vi "Get Result.vi"(8 "error in (no error)":errorcluster, 11 "Keithley Meter in":refnum<class "Keithley Meter.lvclass">) -> (0 "error out":errorcluster, 2 "Mag Lab Result.lvclass":refnum<class "Mag Lab Result.lvclass">, 3 "Keithley Meter out":refnum<class "Keithley Meter.lvclass">)   [LabVIEW 2015, in "Keithley Meter.lvclass"]
uses:
  Keithley Meter.lvclass
  Mag Lab Result/Mag Lab Result.lvclass
  Mag Lab Hardware.lvclass/Mag Lab Hardware.ctl
  Mag Lab Root/Mag Lab Root.lvclass/Mag Lab Root.ctl
  Keithley Meter.lvclass/Keithley Meter.ctl
  Instruments/Keithley/Meter/Keithley Meter Parameters.ctl
  Instruments/Keithley/Meter/KeithleyMeter Function.ctl
  Mag Lab Properties/Mag Lab Parameters.lvclass
  Mag Lab Hardware.lvclass
  Mag Lab Error Handler/Mag Lab Error Handler.lvclass
  Mag Lab Root/Mag Lab Root.lvclass
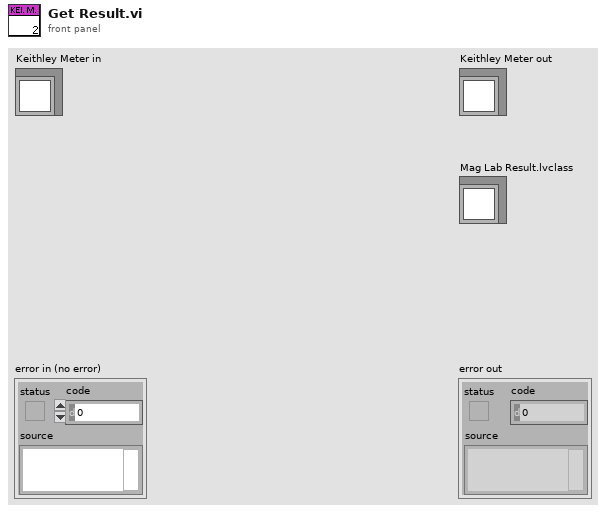
[diagram p1: front panel]
types:
  T1 = typedef "Keithley Meter Parameters.ctl" = cluster{"Range (-1: auto)":dbl, "Integration Time (NPLCs)":dbl, "Function":T2, "W Offset comp":bool, "4-wire W":bool, "Scale":dbl, "Offset":dbl}
  T2 = typedef "KeithleyMeter Function.ctl" = enum16{"VOLTAGE", "CURRENT", "RESISTANCE"}
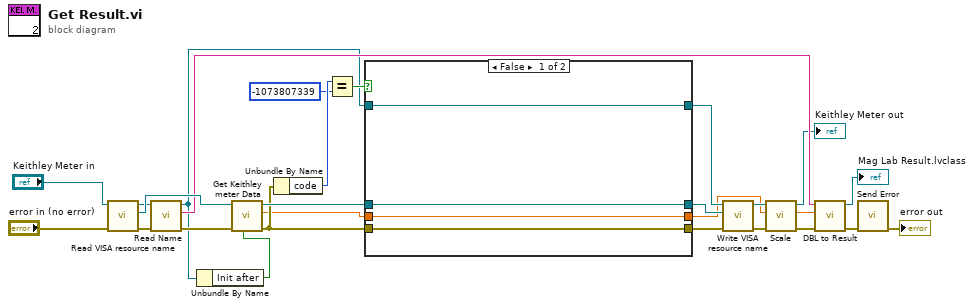
[diagram p0: block diagram]
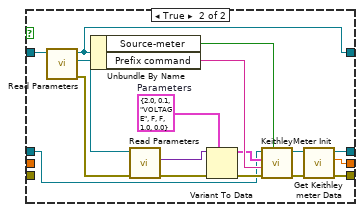
[diagram p2: hidden frame]
diagram:
  n1 = call "Read VISA resource name.vi"("error in (no error)"="error in (no error)", "Mag Lab Hardware in"="Keithley Meter in") -> ("error out"=w24:errorcluster, "VISA resource name"=w26:refnum<visa-resource-name>, "Mag Lab Hardware out"=w25:refnum<class "Keithley Meter.lvclass">)  [unwired: 7 in]
  n2 = call "Read Name.vi"("error in (no error)"=w24, "Mag Lab Root in"=w25) -> ("error out"=w23:errorcluster, "Name"=w19:string, "Mag Lab Root out"=w2:refnum<class "Keithley Meter.lvclass">)  [unwired: 7 in]
  n3 = Unbundle By Name(w2) -> ("Init after"=w1:bool)
  n4 = call "Get Keithley meter Data.vi"("INIT after?"=w1, "error in (no error)"=w23, "VISA Resource Name"=w26) -> ("error out"=w6:errorcluster, "Data"=w3:dbl, "VISA Resource Name Out"=w9:refnum<visa-resource-name>)  [unwired: 6 in]
  n5 = Unbundle By Name(w6) -> ("code"=w12:i32)
  n6 = Equal?(x=w12, y=-1073807339 ("code")) -> (x = y?=w10:bool)
  n7 = case shown="False" w10 {
    tunnel: w2 -> [w29 w39]
    tunnel: w9 -> [w31 w41]
    tunnel: [w31 w34] -> w8
    tunnel: [w30 w33] -> w7
    tunnel: w6 -> [w30 _]
    tunnel: [w29 w38] -> w5
    tunnel: [w28 w32] -> w4
    tunnel: w3 -> [w28 _]
    frame False {
    }
    frame True {
      w47 = T1 {"Range (-1: auto)"=2.0, "Integration Time (NPLCs)"=0.1, "Function"=enum."VOLTAGE", "W Offset comp"=FALSE, "4-wire W"=FALSE, "Scale"=1.0, "Offset"=0.0}  # Parameters
      n8 = call-dynamic "Read Parameters.vi"("Mag Lab Root in"=w39) -> ("error out"=w40:errorcluster, "Mag Lab Parameters.lvclass"=w37:refnum<class "Mag Lab Parameters.lvclass">, "Mag Lab Root out"=w38:refnum<class "Keithley Meter.lvclass">)  [unwired: 8 in]
      n9 = Unbundle By Name(w38) -> ("Source-meter"=w42:bool, "Prefix command"=w48:string)
      n10 = call-dynamic "Read Parameters.vi"("error in (no error)"=w40, "Mag Lab Parameters in"=w37) -> ("error out"=w45:errorcluster, "Parameters"=w46:variant)  [unwired: 7 in, 1 out]
      n11 = Variant To Data(error in=w45, type=w47, Variant=w46) -> (data=w44:T1, error out=w43:errorcluster)
      n12 = call "KeithleyMeter Init.vi"("Source-meter"=w42, "Error In"=w43, "Prefix command"=w48, "Parameters"=w44, "VISA resource name"=w41) -> ("Error Out"=w36:errorcluster, "VISA resource name out"=w35:refnum<visa-resource-name>)  [unwired: 5 in]
      n13 = call "Get Keithley meter Data.vi"("error in (no error)"=w36, "VISA Resource Name"=w35) -> ("error out"=w33:errorcluster, "Data"=w32:dbl, "VISA Resource Name Out"=w34:refnum<visa-resource-name>)  [unwired: 7 in]
    }
  }
  n14 = call "Write VISA resource name.vi"("error in (no error)"=w7, "VISA resource name"=w8, "Mag Lab Hardware in"=w5) -> ("error out"=w13:errorcluster, "Mag Lab Hardware out"=w22:refnum<class "Keithley Meter.lvclass">)  [unwired: 7 in]
  n15 = call-dynamic "Scale.vi"("error in (no error)"=w13, "Input"=w4, "Meter in"=w22) -> ("error out"=w14:errorcluster, "Output"=w15:dbl, "Meter out"=→"Keithley Meter out":refnum<class "Keithley Meter.lvclass">)  [unwired: 6 in]
  n16 = call "DBL to Result.vi"("error in (no error)"=w14, "Data"=w15, "Name"=w19) -> ("error out"=w18:errorcluster, "Mag Lab Result out"=→"Mag Lab Result.lvclass":refnum<class "Mag Lab Result.lvclass">)  [unwired: 7 in]
  n17 = call "Send Error.vi"("error in (no error)"=w18) -> ("error out"=→"error out":errorcluster)  [unwired: 9 in, 1 out]
